vi "JedanMotor_host_DrajverStari.vi"() -> ()   [LabVIEW 2014]
uses:
  <vilib>/FPGAPlugInAG/sbRIO-9636/niLvFpga_Open_sbRIO-9636.vi
  <vilib>/rvi/interface/common/dynamic/niFpgaDynamicAddResources.vi
  <vilib>/Utility/error.llb/Error Cluster From Error Code.vi
  <vilib>/rvi/errors/niLvFpgaAdjustHostInterfaceError.vi
  <vilib>/FPGAPlugInAG/Dynamic/niLvFpga_Close_Dynamic.vi
  <vilib>/rvi/interface/nirviOpenFPGA/nirviOpenFPGA.xnode
  FPGA Bitfiles/JedanMotorDrajve_FPGATarget_JedanMotorfpgaDr_Xg6zrhxYVYA.lvbitx
  <vilib>/rvi/interface/nirviReadWriteControl/nirviReadWriteControl.xnode
  <vilib>/rvi/interface/nirviCloseFPGA/nirviCloseFPGA.xnode
  NiFpgaLv.dll
  <vilib>/rvi/interface/Simulation/niFpgaSimulationCallBeginRW.vi
panel:
  in  "direction":fxp<+/-,64,32>
  in  "Step":sgl(knob) scale=0.0..300.0
  in  "MS3":bool
  in  "MS2":bool
  in  "MS1":bool
  in  "stop":bool
  # "Izabri koraèni mod:"
  # "Izaberi brzinu motora:"
  # "Zaustavi motor:"
  # "Izaberi smjer kretanja (naprijed/nazad):"
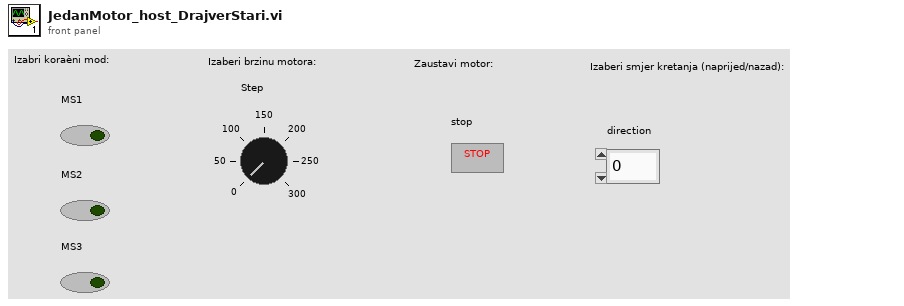
[diagram p1: front panel]
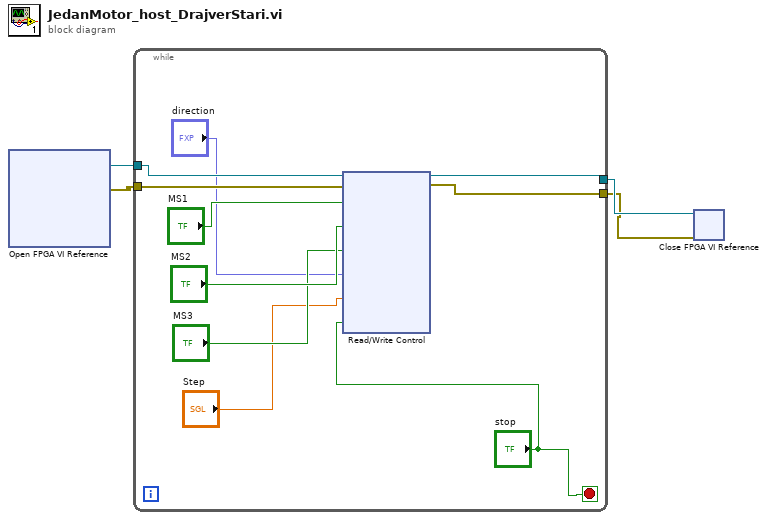
[diagram p0: block diagram]
diagram:
  n1 = xnode "Open FPGA VI Reference"() -> ("FPGA VI Reference Out"=w4:refnum<k20>, "error out"=w3:errorcluster)  [unwired: 2 in]
  n2 = while {
    tunnel: w4 -> [w14]
    tunnel: w3 -> [w13]
    tunnel: [w12] -> w2
    tunnel: [w11] -> w1
    stop <- "stop" stop-if-true
    n3 = xnode "Read/Write Control"("FPGA VI Reference In"=w14, "error in"=w13, "MS1"="MS1", "MS2"="MS2", "MS3"="MS3", "direction"="direction", "step"="Step", "stop"="stop") -> ("FPGA VI Reference Out"=w12:refnum<k20>, "error out"=w11:errorcluster)
  }
  n4 = xnode "Close FPGA VI Reference"("FPGA VI Reference In"=w2, "error in"=w1) -> ()  [unwired: 1 out]
